vi "7_segment_display.vi"() -> ()   [LabVIEW 2019]
panel:
  in  "Numeric":u8=6
  in  "Button":bool
  out "f":bool
  out "e":bool
  out "d":bool
  out "c":bool
  out "g":bool
  out "b":bool
  out "a":bool
  # "7 segment dispay"
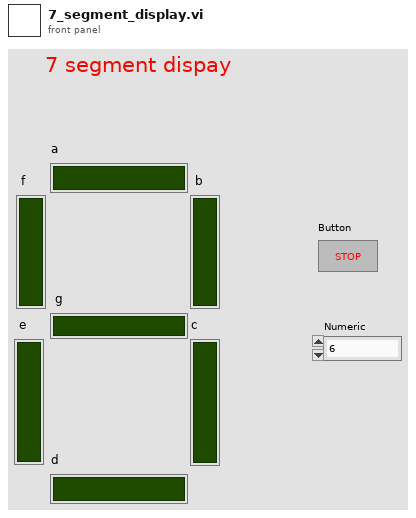
[diagram p1: front panel]
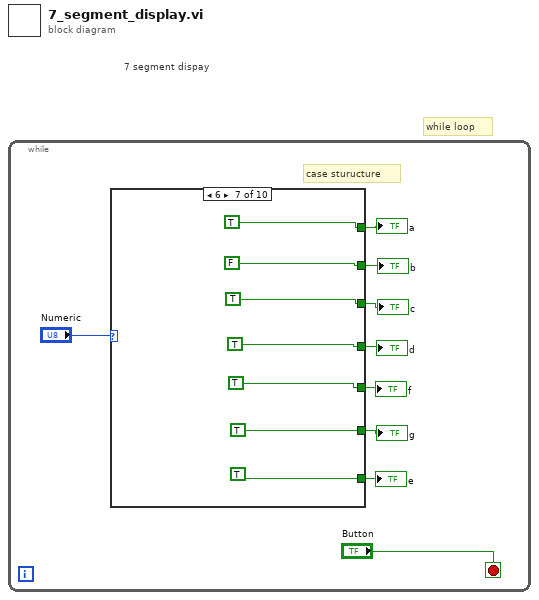
[diagram p0: block diagram]
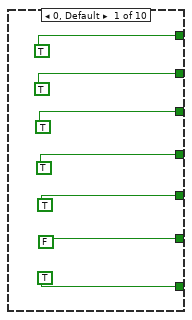
[diagram p2: hidden frame]
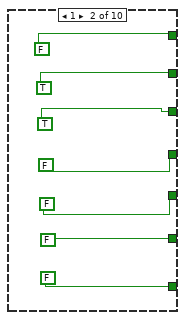
[diagram p3: hidden frame]
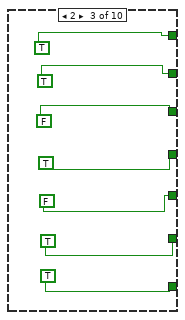
[diagram p4: hidden frame]
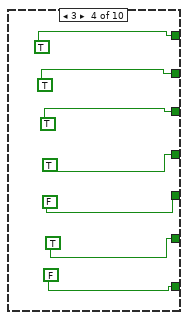
[diagram p5: hidden frame]
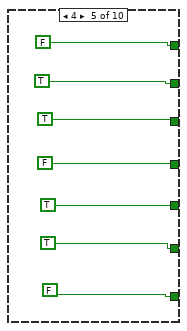
[diagram p6: hidden frame]
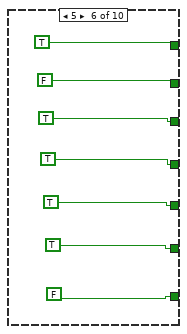
[diagram p7: hidden frame]
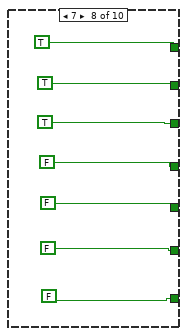
[diagram p8: hidden frame]
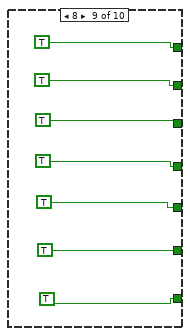
[diagram p9: hidden frame]
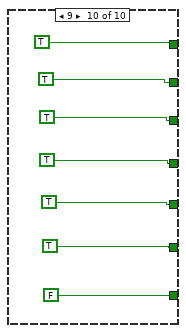
[diagram p10: hidden frame]
diagram:
  # "while loop"
  # "7 segment dispay"
  n1 = while {
    stop <- "Button" stop-if-true
    # "case sturucture"
    n2 = case shown="6" "Numeric" {
      tunnel: [TRUE FALSE TRUE TRUE FALSE TRUE TRUE TRUE TRUE TRUE] -> w7
      tunnel: [TRUE TRUE TRUE TRUE TRUE FALSE FALSE TRUE TRUE TRUE] -> w6
      tunnel: [TRUE FALSE TRUE TRUE FALSE TRUE TRUE FALSE TRUE TRUE] -> w5
      tunnel: [TRUE FALSE FALSE FALSE TRUE TRUE TRUE FALSE TRUE TRUE] -> w4
      tunnel: [FALSE FALSE TRUE TRUE TRUE TRUE TRUE FALSE TRUE TRUE] -> w3
      tunnel: [TRUE FALSE TRUE FALSE FALSE FALSE TRUE FALSE TRUE FALSE] -> w2
      tunnel: [TRUE TRUE FALSE TRUE TRUE TRUE TRUE TRUE TRUE TRUE] -> w1
      frame 0, Default {
      }
      frame 1 {
      }
      frame 2 {
      }
      frame 3 {
      }
      frame 4 {
      }
      frame 5 {
      }
      frame 6 {
      }
      frame 7 {
      }
      frame 8 {
      }
      frame 9 {
      }
    }
    "a" <- w7
    "b" <- w6
    "g" <- w3
    "c" <- w1
    "d" <- w5
    "e" <- w2
    "f" <- w4
  }
